vi "Get Injected Value static.vi"(8 "error in (no error)":errorcluster, 11 "Fault-Injection_DBL in":refnum<class "Fault-Injection_STR.lvclass">) -> (0 "error out":errorcluster, 2 "Value":T1, 3 "Fault-Injection_DBL out":refnum<class "Fault-Injection_STR.lvclass">)   [LabVIEW 2021, in "Fault-Injection_STR.lvclass"]
uses:
  Fault-Injection_STR.lvclass
  Value Type.ctl
  Fault-Injection_STR.lvclass/Fault-Injection_STR.ctl
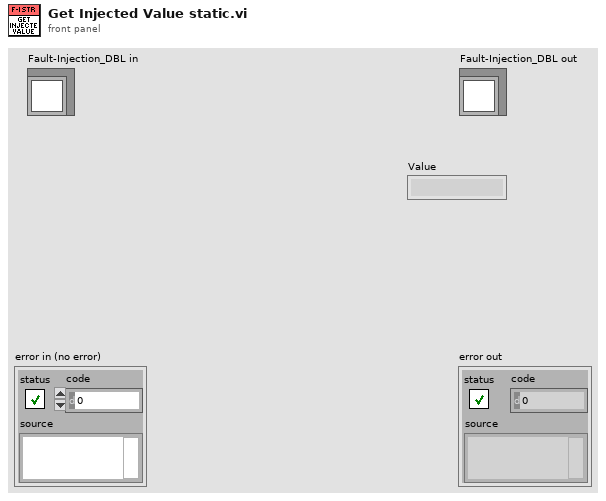
[diagram p1: front panel]
types:
  T1 = typedef "Fault-Injection_STR.lvclass/Value Type.ctl" = string
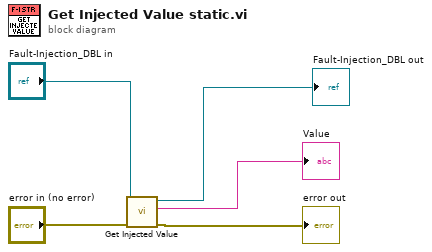
[diagram p0: block diagram]
diagram:
  n1 = call-dynamic "Get Injected Value.vi"("error in (no error)"="error in (no error)", "Fault-Injection_Boolean in"="Fault-Injection_DBL in") -> ("error out"=→"error out":errorcluster, "Value"=→"Value":T1, "Fault-Injection_Boolean out"=→"Fault-Injection_DBL out":refnum<class "Fault-Injection_STR.lvclass">)  [unwired: 7 in]
